vi "PlotSine.vi"() -> ()   [LabVIEW 2020]
panel:
  in  "Numeric":i32
  out "Mixed Signal Graph":dbl[][](graph)
  out "Waveform Graph 3":dbl[](graph)
  in  "x 3":dbl
  in  "x":dbl
  out "Waveform Graph":dbl[](graph)
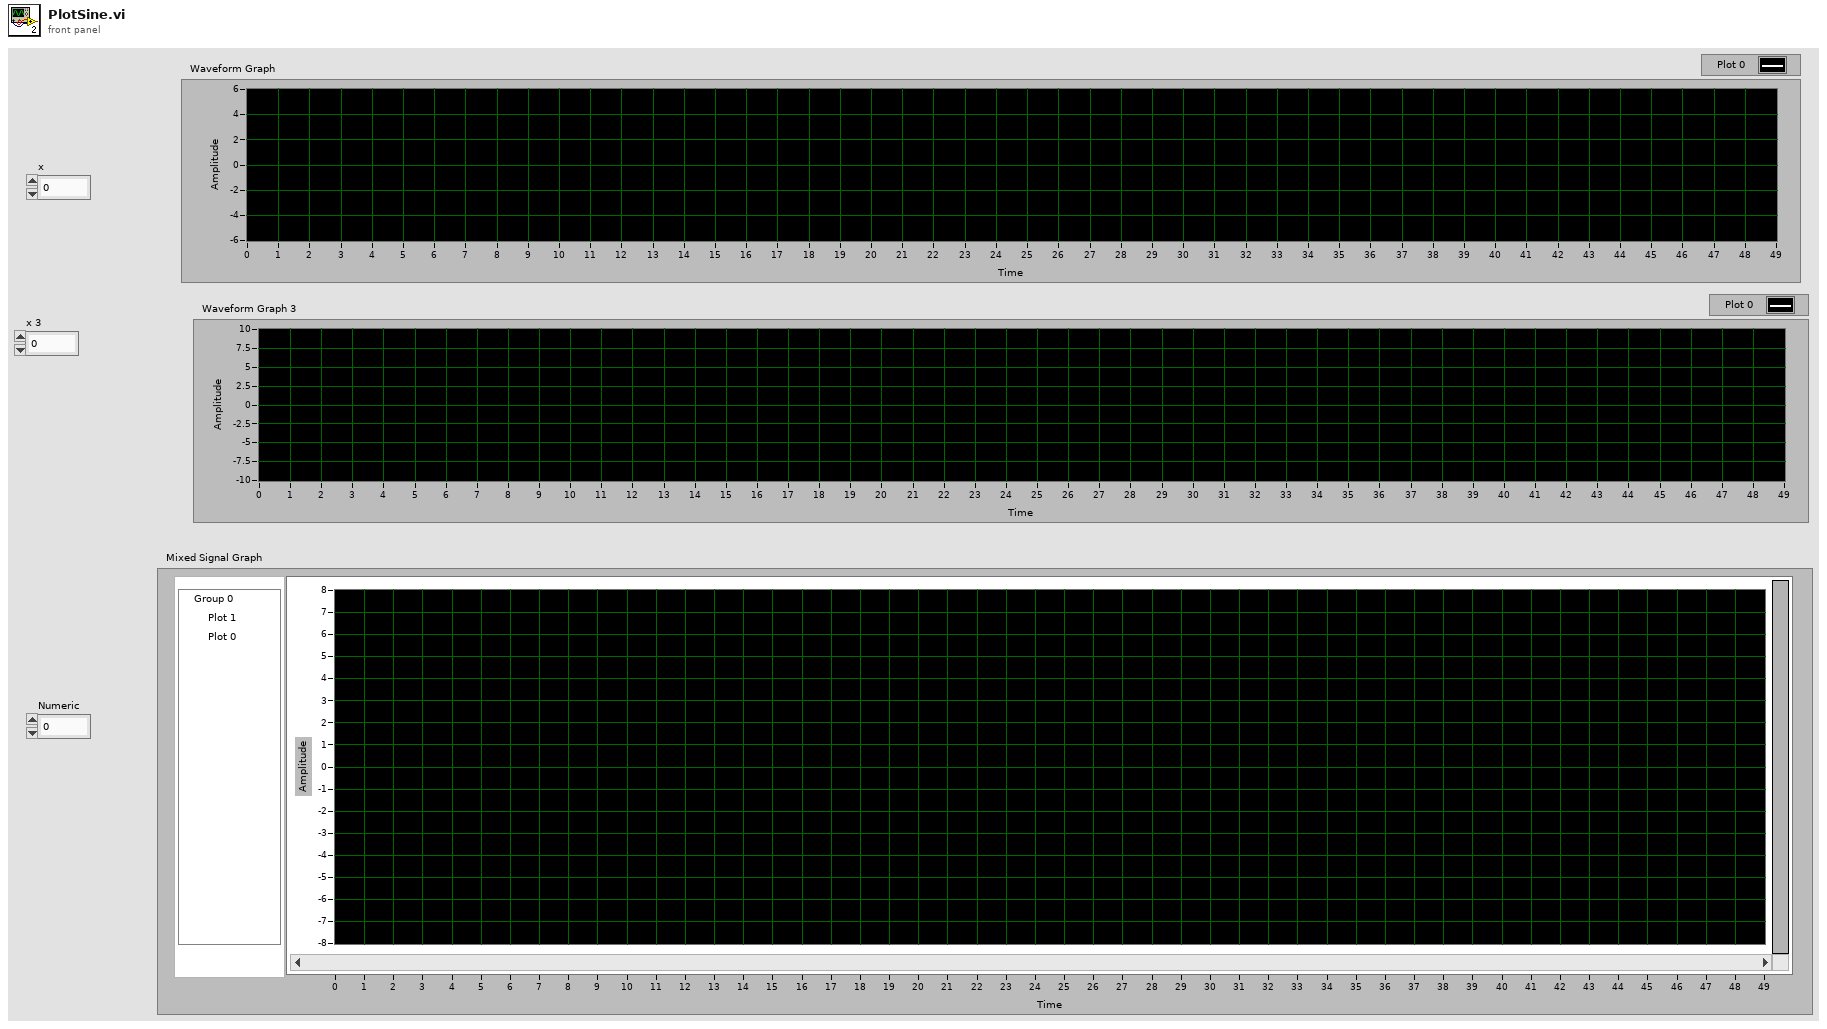
[diagram p1: front panel]
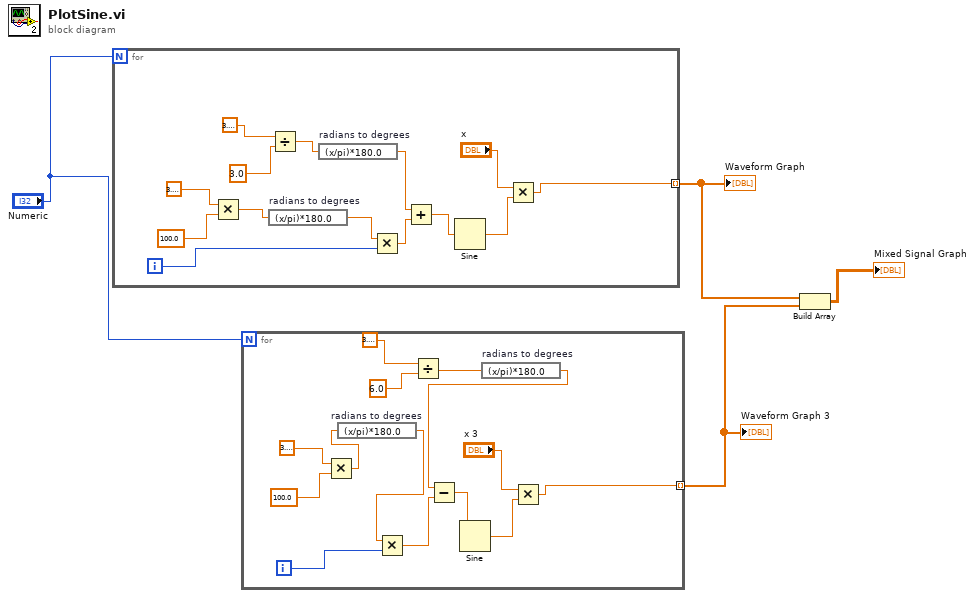
[diagram p0: block diagram]
diagram:
  n1 = for {
    N: "Numeric" -> [_]
    tunnel: [w10] -> w4 mode=indexing
    i -> [w11]
    n2 = Multiply(x=3.141592653589793, y=100.0 ("x")) -> (x*y=w8:dbl)
    n3 = expression code="(x/pi)*180.0" "radians to degrees"(w8) -> (w7:dbl)
    n4 = Divide(x=3.141592653589793, y=3.0) -> (x/y=w6:dbl)
    n5 = expression code="(x/pi)*180.0" "radians to degrees"(w6) -> (w5:dbl)
    n6 = Multiply(x=w7, y=w11) -> (x*y=w14:dbl)
    n7 = Add(x=w5, y=w14) -> (x+y=w13:dbl)
    n8 = Sine(x=w13) -> (sin(x)=w12:dbl)
    n9 = Multiply(x="x", y=w12) -> (x*y=w10:dbl)
  }
  "Waveform Graph" <- w4
  n10 = for {
    N: "Numeric" -> [_]
    tunnel: [w30] -> w3 mode=indexing
    i -> [w31]
    n11 = Multiply(x=3.141592653589793, y=100.0 ("x")) -> (x*y=w26:dbl)
    n12 = expression code="(x/pi)*180.0" "radians to degrees"(w26) -> (w25:dbl)
    n13 = Multiply(x=w25, y=w31) -> (x*y=w20:dbl)
    n14 = Divide(x=3.141592653589793, y=6.0) -> (x/y=w22:dbl)
    n15 = expression code="(x/pi)*180.0" "radians to degrees"(w22) -> (w19:dbl)
    n16 = Subtract(x=w19, y=w20) -> (x-y=w21:dbl)
    n17 = Sine(x=w21) -> (sin(x)=w32:dbl)
    n18 = Multiply(x="x 3", y=w32) -> (x*y=w30:dbl)
  }
  "Waveform Graph 3" <- w3
  n19 = Build Array(w4, w3) -> (→"Mixed Signal Graph":dbl[][])
